vi "FPGA Main.vi"() -> ()   [LabVIEW 2018]
uses:
  Program Files (x86)/National Instruments/LabVIEW 2018/ProjectTemplates/Source/myRIO/Oscilloscope/myRIO v1.1/Real-Time/Controls/Wave Properties - FPGA.ctl
  Program Files (x86)/National Instruments/LabVIEW 2018/ProjectTemplates/Source/myRIO/Oscilloscope/myRIO v1.1/Real-Time/Controls/Waveform Enum.ctl
  Program Files (x86)/National Instruments/LabVIEW 2018/ProjectTemplates/Source/myRIO/Oscilloscope/myRIO v1.1/Real-Time/Controls/Channel Selector.ctl
  <vilib>/rvi/Emulation/niFpgaGetClockAttributes.vi
  <vilib>/rvi/Emulation/niFpgaSctlEmulationGetInTimedLoop.vi
  <vilib>/rvi/Emulation/niFpgaEmulationReportErrorSimple.vi
  <vilib>/rvi/eio/common/nirviEmuTemplateMethod_errors.vi
  <vilib>/rvi/Emulation/niFpgaCriticalErrorInLSC.vi
  <vilib>/rvi/interface/RandomDataEmulation/niFpgaRandomDataHandleErrors.vi
  <vilib>/eio/EIONode/EIONode.xnode
  <vilib>/rvi/DataTransferAndStorage/Container/XNode/niFpgaContainer.xnode
  <vilib>/rvi/interface/RandomDataEmulation/nirviRandomDataFpgaReadWriteTemplate.vi
panel:
  in  "Stop Output 2":bool
  in  "Initialize AO1":bool
  in  "Wave Properties AO1":T1
  out "Actual loop rate (AO1)":u32=1000
  in  "AO1 Loop Rate (ticks)":u32=1000
  in  "Wave Properties AO0":T1
  out "Actual loop rate (Acq)":u32=1000
  out "ConnectorC/AI1":i16
  out "ConnectorC/AI0":i16
  in  "Acq Rate(ticks)":u32 caption="Acq Rate(us)"
  in  "Stop Input":bool
  in  "Stop Output":bool
  in  "Initialize AO0":bool
  out "Actual loop rate (AO0)":u32=1000
  in  "AO0 Loop Rate (ticks)":u32=1000
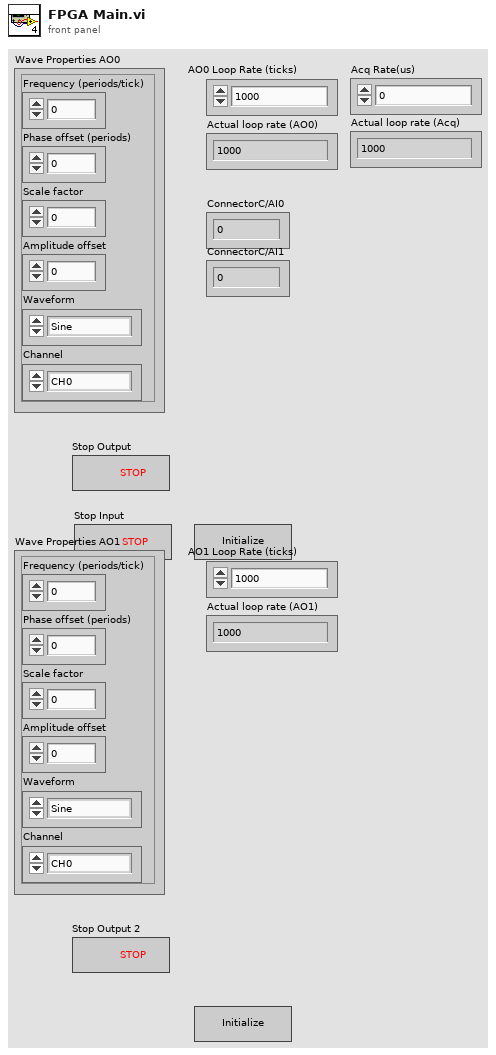
[diagram p1: front panel]
types:
  T1 = typedef "Wave Properties - FPGA.ctl" = cluster{"Frequency (periods/tick)":fxp<+,32,0>, "Phase offset (periods)":fxp<+,32,0>, "Scale factor":fxp<+/-,24,1>, "Amplitude offset":fxp<+/-,24,12>, "Waveform":T2, "Channel":T3}
  T2 = typedef "Waveform Enum.ctl" = enum16{"Sine", "Square"}
  T3 = typedef "Channel Selector.ctl" = enum16{"CH0", "CH1"}
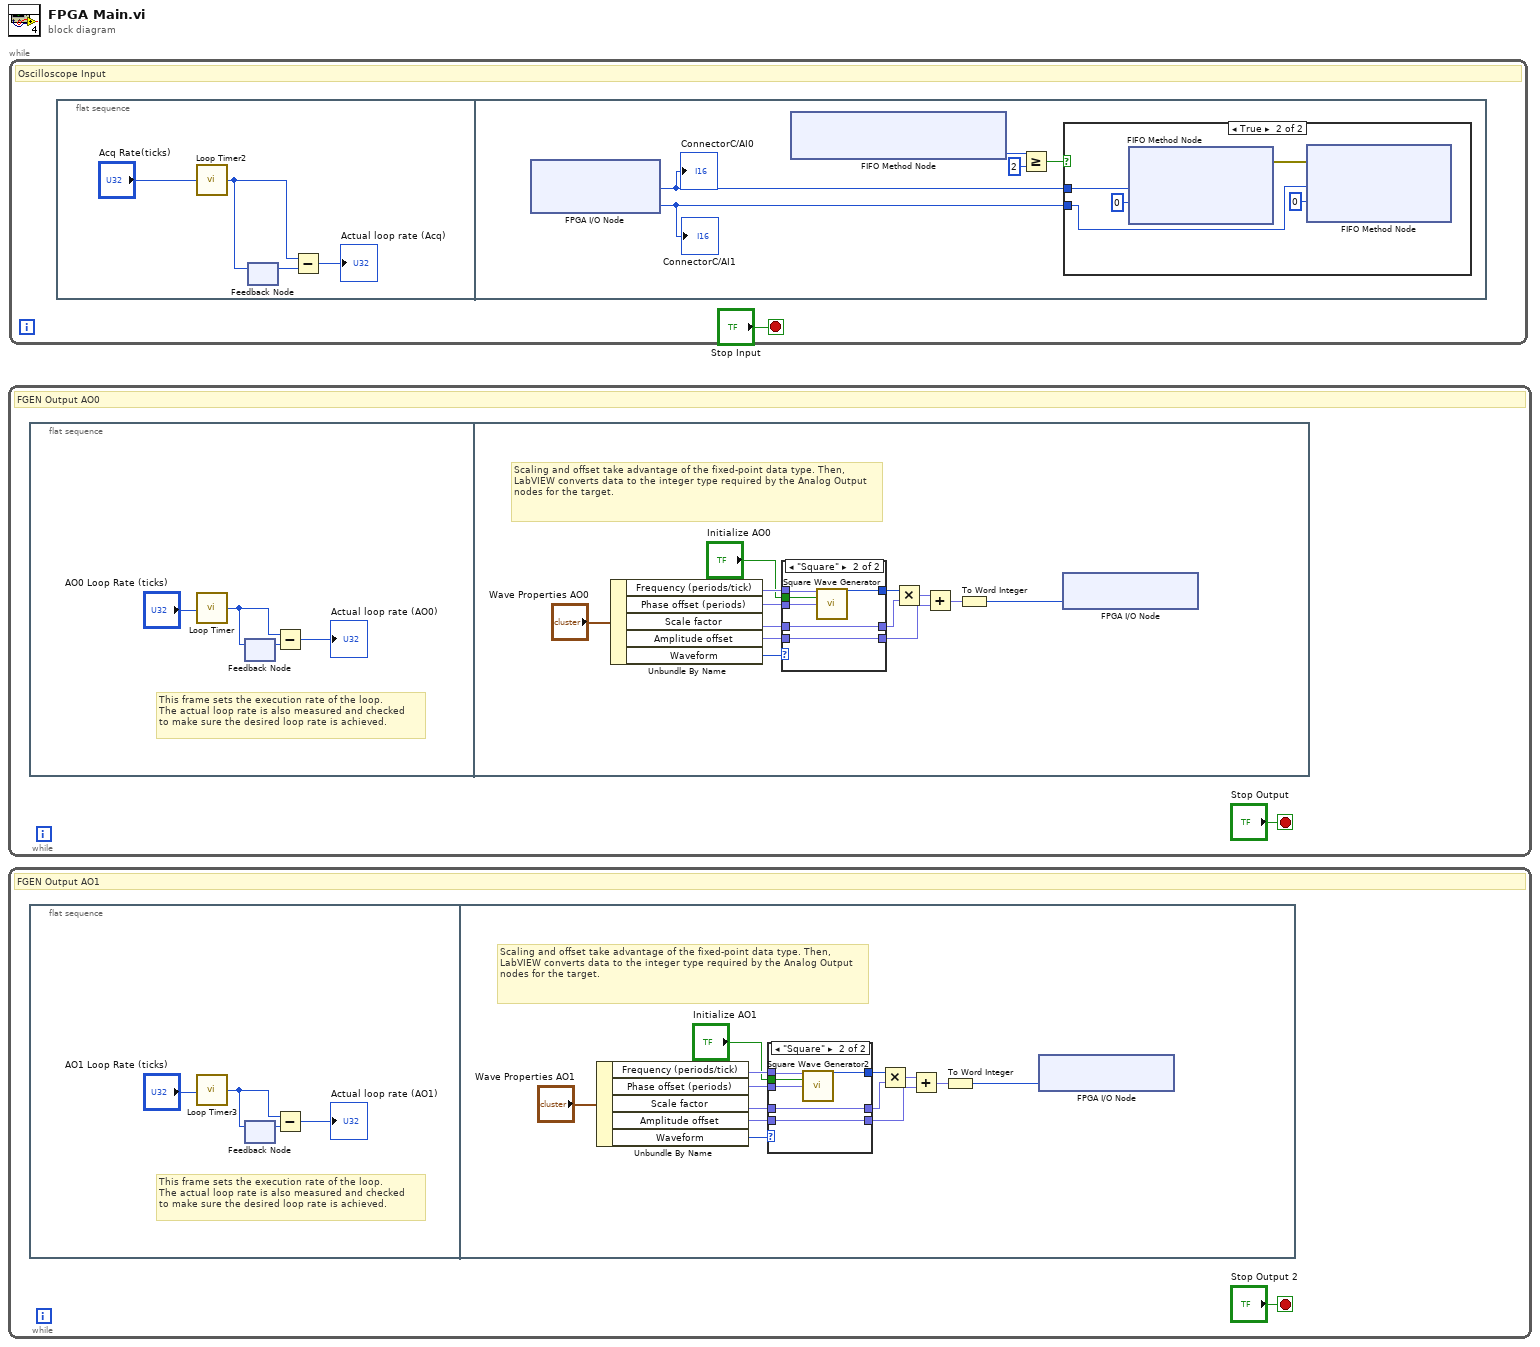
[diagram p0: block diagram]
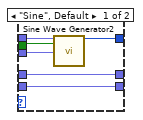
[diagram p2: hidden frame]
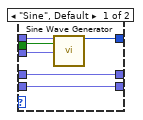
[diagram p4: hidden frame]
diagram:
  n1 = while {
    stop <- "Stop Output" stop-if-true
    # "FGEN Output AO0"
    n2 = flat-sequence {
      frame #0 {
        # "This frame sets the execution rate of the loop.\nThe actual loop rate is also measured and checked\nto make sure the desired loop rate is achieved."
        n3 = call "Loop Timer"("Count(Ticks)"="AO0 Loop Rate (ticks)") -> ("Tick Count(Ticks)"=w3:u32)
        n4 = feedback-in #1(w3) -> ()
        n5 = feedback #1() -> (w4:u32)  [unwired: 1 out]
        n6 = Subtract(x=w3, y=w4) -> (x-y=→"Actual loop rate (AO0)":u32)
      }
      frame #1 {
        # "Scaling and offset take advantage of the fixed-point data type. Then, LabVIEW converts data to the integer type required by the Analog Output nodes for the target."
        n7 = Unbundle By Name("Wave Properties AO0") -> ("Frequency (periods/tick)"=w18:fxp<+,32,0>, "Phase offset (periods)"=w17:fxp<+,32,0>, "Scale factor"=w15:fxp<+/-,24,1>, "Amplitude offset"=w14:fxp<+/-,24,12>, "Waveform"=w8:T2)
        n8 = case shown="\"Square\"" w8 {
          tunnel: w18 -> [w24 w30]
          tunnel: w17 -> [w23 w28]
          tunnel: "Initialize AO0" -> [w22 w29]
          tunnel: [w21 w25] -> w13
          tunnel: w15 -> [w20 w27]
          tunnel: [w20 w27] -> w12
          tunnel: w14 -> [w19 w26]
          tunnel: [w19 w26] -> w10
          frame "Sine", Default {
            n9 = call "Sine Wave Generator"("frequency (periods/tick)"=w24, "reset"=w22, "phase offset (periods)"=w23) -> ("sine out"=w21:i16)  [unwired: 12 in]
          }
          frame "Square" {
            n10 = call "Square Wave Generator"("frequency (periods/tick)"=w30, "reset"=w29, "phase offset (periods)"=w28) -> ("square wave out"=w25:i16)  [unwired: 12 in]
          }
        }
        n11 = Multiply(x=w13, y=w12) -> (x*y=w11:fxp<+/-,40,17>)
        n12 = Add(x=w11, y=w10) -> (x+y=w9:fxp<+/-,40,17>)
        n13 = To Word Integer(number=w9) -> (16bit integer=w7:i16)
        n14 = xnode "FPGA I/O Node"("ConnectorC/AO0"=w7) -> ()  [unwired: 1 in, 1 out]
      }
    }
  }
  n15 = while {
    stop <- "Stop Output 2" stop-if-true
    # "FGEN Output AO1"
    n16 = flat-sequence {
      frame #0 {
        # "This frame sets the execution rate of the loop.\nThe actual loop rate is also measured and checked\nto make sure the desired loop rate is achieved."
        n17 = call "Loop Timer3"("Count(Ticks)"="AO1 Loop Rate (ticks)") -> ("Tick Count(Ticks)"=w33:u32)
        n18 = feedback-in #2(w33) -> ()
        n19 = feedback #2() -> (w34:u32)  [unwired: 1 out]
        n20 = Subtract(x=w33, y=w34) -> (x-y=→"Actual loop rate (AO1)":u32)
      }
      frame #1 {
        # "Scaling and offset take advantage of the fixed-point data type. Then, LabVIEW converts data to the integer type required by the Analog Output nodes for the target."
        n21 = Unbundle By Name("Wave Properties AO1") -> ("Frequency (periods/tick)"=w48:fxp<+,32,0>, "Phase offset (periods)"=w47:fxp<+,32,0>, "Scale factor"=w45:fxp<+/-,24,1>, "Amplitude offset"=w44:fxp<+/-,24,12>, "Waveform"=w38:T2)
        n22 = case shown="\"Square\"" w38 {
          tunnel: w48 -> [w54 w60]
          tunnel: w47 -> [w53 w58]
          tunnel: "Initialize AO1" -> [w52 w59]
          tunnel: [w51 w55] -> w43
          tunnel: w45 -> [w50 w57]
          tunnel: [w50 w57] -> w42
          tunnel: w44 -> [w49 w56]
          tunnel: [w49 w56] -> w40
          frame "Sine", Default {
            n23 = call "Sine Wave Generator2"("frequency (periods/tick)"=w54, "reset"=w52, "phase offset (periods)"=w53) -> ("sine out"=w51:i16)  [unwired: 12 in]
          }
          frame "Square" {
            n24 = call "Square Wave Generator2"("frequency (periods/tick)"=w60, "reset"=w59, "phase offset (periods)"=w58) -> ("square wave out"=w55:i16)  [unwired: 12 in]
          }
        }
        n25 = Multiply(x=w43, y=w42) -> (x*y=w41:fxp<+/-,40,17>)
        n26 = Add(x=w41, y=w40) -> (x+y=w39:fxp<+/-,40,17>)
        n27 = To Word Integer(number=w39) -> (16bit integer=w37:i16)
        n28 = xnode "FPGA I/O Node"("ConnectorC/AO1"=w37) -> ()  [unwired: 1 in, 1 out]
      }
    }
  }
  n29 = while {
    stop <- "Stop Input" stop-if-true
    # "Oscilloscope Input"
    n30 = flat-sequence {
      frame #0 {
        n31 = call "Loop Timer2"("Count(Ticks)"="Acq Rate(ticks)") -> ("Tick Count(Ticks)"=w62:u32)
        n32 = feedback #3() -> (w63:u32)  [unwired: 1 out]
        n33 = feedback-in #3(w62) -> ()
        n34 = Subtract(x=w62, y=w63) -> (x-y=→"Actual loop rate (Acq)":u32)
      }
      frame #1 {
        n35 = xnode "FPGA I/O Node"() -> ("ConnectorC/AI0"=w67:i16, "ConnectorC/AI1"=w66:i16)  [unwired: 2 in, 2 out]
        "ConnectorC/AI0" <- w67
        "ConnectorC/AI1" <- w66
        n36 = xnode ("FIFO Method Node")() -> ("Number of Elements to Write"=w68:u32)  [unwired: 1 in, 1 out]
        n37 = Greater Or Equal?(x=w68, y=u32 2) -> (x >= y?=w70:bool)
        n38 = case shown="True" w70 {
          tunnel: w67 -> [_ w73]
          tunnel: w66 -> [_ w72]
          frame False {
          }
          frame True {
            n39 = xnode ("FIFO Method Node")("Element"=w73, "Timeout"=0) -> ("error out"=w74:errorcluster)  [unwired: 2 in, 2 out]
            n40 = xnode ("FIFO Method Node")("Element"=w72, "Timeout"=0, "error in (no error)"=w74) -> ()  [unwired: 1 in, 3 out]
          }
        }
      }
    }
  }
